vi "XML_FAIL.vi"(10 "SerialNumber":string, 11 "StatusCode":string) -> (2 "字符串":string, 3 "字符串 2":string)   [LabVIEW 2018]
uses:
  Subvi/Global.vi
panel:
  # "2021-04-17T10:09:51"
  # "2021-4-28T10:29:08"
  # "<Unit Timestamp=\"2021-04-17T10:09:51\" SerialNumber=\"KF1118M4A00643\" DateTimeStart=\"2021-04-17T10:09:39\" DateTimeEnd=\"2021-04-17T10:09:51\" xmlns=\"Valor.vCheckTester.xsd\" StatusCode=\"PASS\">"
  # "<Header TestProgramName=\"HW\" TestHeadNumber=\"HW\" TestProgramVersion=\"V1.0.0\" TestHeadType=\"Testser Information\" TestFixtureNumber=\"00001\"/>\n</Unit>\n</vCheckTester>"
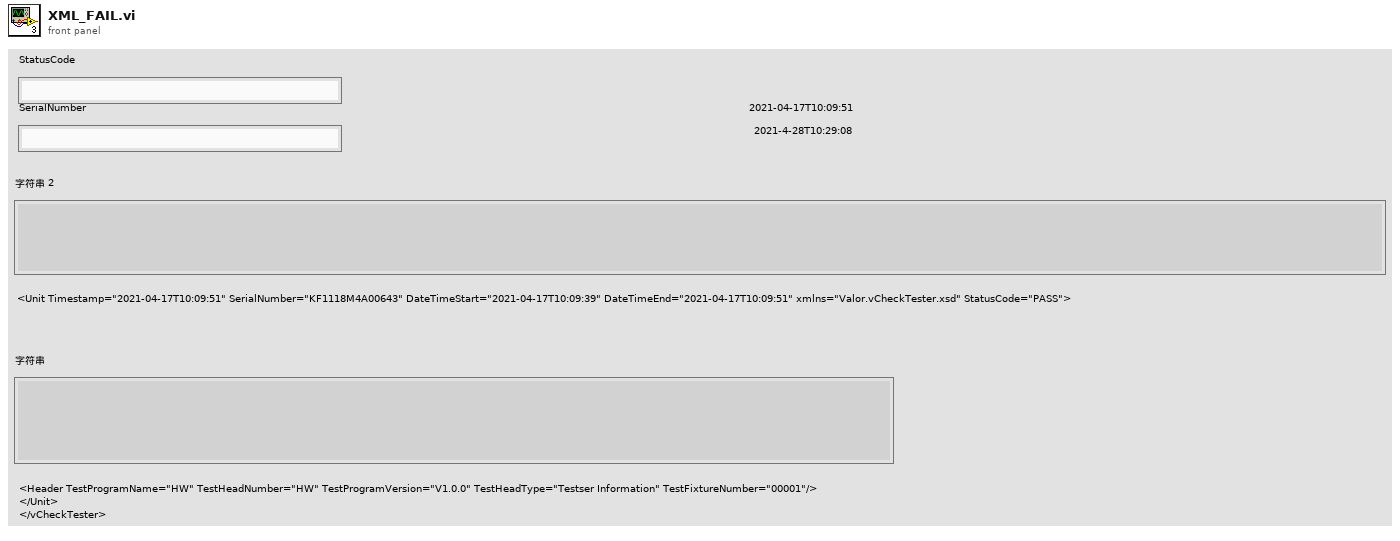
[diagram p1: front panel]
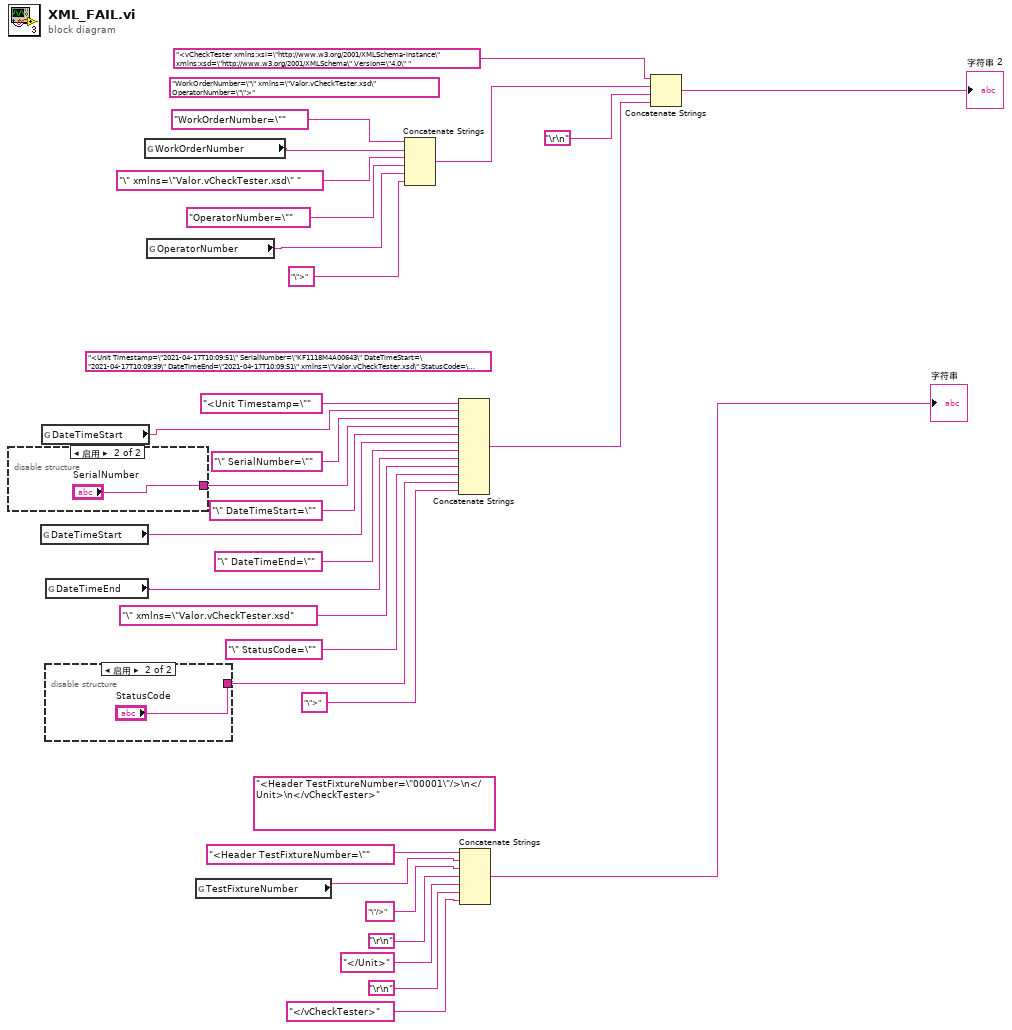
[diagram p0: block diagram]
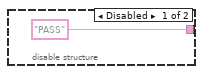
[diagram p2: hidden frame]
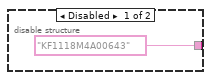
[diagram p3: hidden frame]
diagram:
  (unwired) "<Header TestFixtureNumber=\"00001\"/>\n</Unit>\n</vCheckTester>"
  (unwired) "<Unit Timestamp=\"2021-04-17T10:09:51\" SerialNumber=\"KF1118M4A00643\" DateTimeStart=\"2021-04-17T10:09:39\" DateTimeEnd=\"2021-04-17T10:09:51\" xmlns=\"Valor.vCheckTester.xsd\" StatusCode=\"PASS\">"
  (unwired) "WorkOrderNumber=\"\" xmlns=\"Valor.vCheckTester.xsd\" OperatorNumber=\"\">"
  n1 = disable-structure shown="启用" {
    disable-tunnel: ["KF1118M4A00643" "SerialNumber"] -> w21
    frame Disabled {
    }
    frame Enabled {
    }
  }
  n2 = global read "Global.vi" "DateTimeStart"() -> (w6:string)
  n3 = global read "Global.vi" "DateTimeStart"() -> (w4:string)
  n4 = global read "Global.vi" "DateTimeEnd"() -> (w5:string)
  n5 = disable-structure shown="启用" {
    disable-tunnel: ["PASS" "StatusCode"] -> w16
    frame Disabled {
    }
    frame Enabled {
    }
  }
  n6 = global read "Global.vi" "WorkOrderNumber"() -> (w2:string)
  n7 = global read "Global.vi" "OperatorNumber"() -> (w1:string)
  n8 = global read "Global.vi" "TestFixtureNumber"() -> (w3:string)
  n9 = Concatenate Strings("WorkOrderNumber=\"", w2, "\" xmlns=\"Valor.vCheckTester.xsd\" ", "OperatorNumber=\"", w1, "\">") -> (w24:string)
  n10 = Concatenate Strings("<Unit Timestamp=\"", w4, "\" SerialNumber=\"", w21, "\" DateTimeStart=\"", w6, "\" DateTimeEnd=\"", w5, "\" xmlns=\"Valor.vCheckTester.xsd", "\" StatusCode=\"", w16, "\">") -> (w14:string)
  n11 = Concatenate Strings("<Header TestFixtureNumber=\"", w3, "\"/>", "\r\n", "</Unit>", "\r\n", "</vCheckTester>") -> (→"字符串":string)
  n12 = Concatenate Strings("<vCheckTester xmlns:xsi=\"http://www.w3.org/2001/XMLSchema-instance\" xmlns:xsd=\"http://www.w3.org/2001/XMLSchema\" Version=\"4.0\" ", w24, "\r\n", w14) -> (→"字符串 2":string)
